vi "Curtin1_AskCal.vi"(9 "Calibration":dbl format="%#g", 11 "Message":string) -> (1 "Calibration out":dbl)   [LabVIEW 2024]
panel:
  in  "Cancel":bool
  in  "OK":bool caption="OK2"
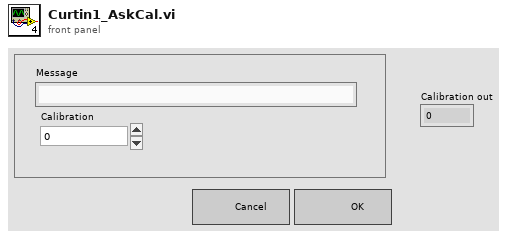
[diagram p1: front panel]
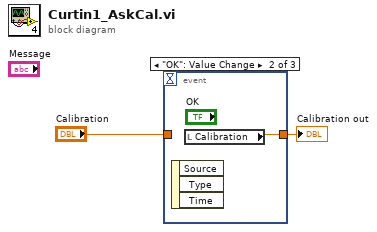
[diagram p0: block diagram]
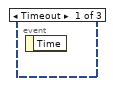
[diagram p2: hidden frame]
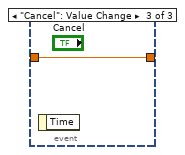
[diagram p3: hidden frame]
diagram:
  n1 = event shown="[1] \"OK\": Value Change" {
    selector: _ -> [_ _ _]
    dyn-events: _ -> [_ _ _]
    timeout: _ -> [_ _ _]
    tunnel: [_ w3 w4] -> w1
    tunnel: "Calibration" -> [_ _ w4]
    event Timeout {
      n2 = event-data() -> ()  [unwired: 1 in, 1 out]
    }
    event "OK": Value Change {
      n3 = event-data() -> ()  [unwired: 1 in, 3 out]
      n4 = local read "Calibration"() -> (w3:dbl)
    }
    event "Cancel": Value Change {
      n5 = event-data() -> ()  [unwired: 1 in, 1 out]
    }
  }
  "Calibration out" <- w1
